vi "gmmregDefaultParameters.vi"(0 "D (3)":i32=3, 1 "nctrlPts":i32=3) -> (2 "param0":dbl[](array[numeric]), 3 "nscales":i32, 4 "default scales":dbl[](array[numeric]), 5 "deault lambdas":dbl[](array[numeric]))   [LabVIEW 2017]
panel:
  in  "lambda":dbl[](array[numeric])
  in  "scales":dbl[](array[numeric])=[1.0, 0.5, 0.1]
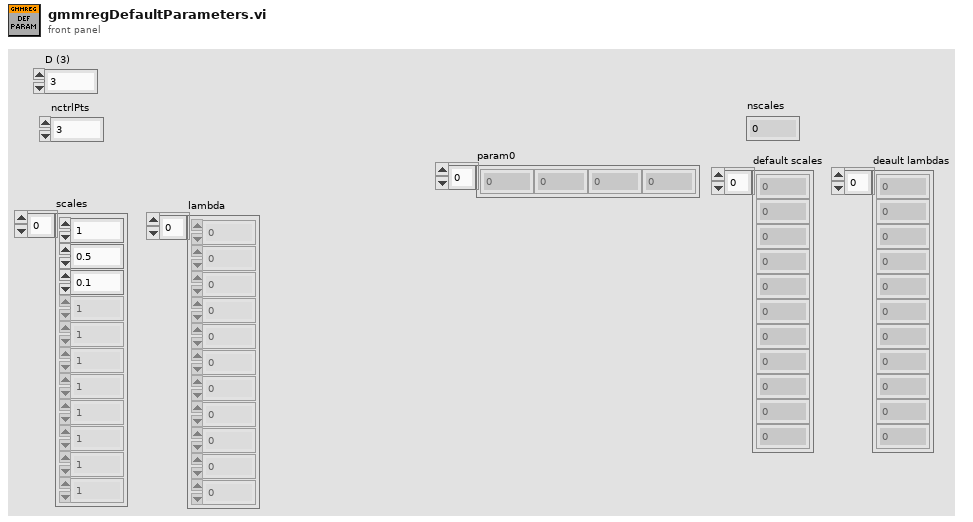
[diagram p1: front panel]
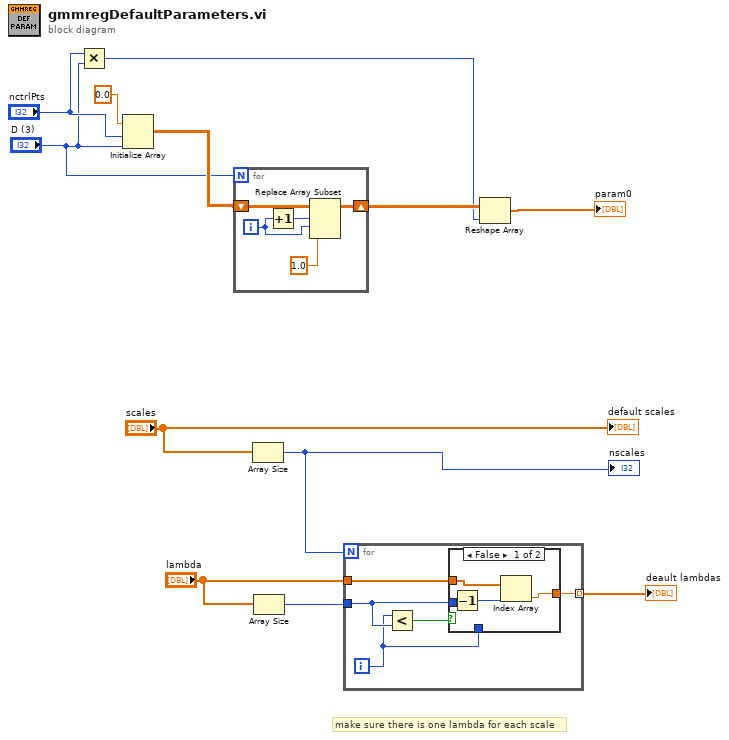
[diagram p0: block diagram]
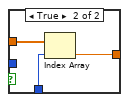
[diagram p2: hidden frame]
diagram:
  # "make sure there is one lambda for each scale"
  n1 = Multiply(x="nctrlPts", y="D (3)") -> (x*y=w2:i32)
  n2 = Initialize Array(0.0 ("element"), "nctrlPts", "D (3)") -> (w11:dbl[][])
  n3 = for {
    N: "D (3)" -> [_]
    shift-right: [w14] -> w5
    shift-left: w11 -> [w13]
    i -> [w16]
    n4 = Increment(x=w16) -> (x+1=w17:i32)
    n5 = Replace Array Subset(array=w13, new element=1.0 ("new element/subarray"), index (row)=w17, index (col)=w16) -> (w14:dbl[][])
  }
  n6 = Array Size(array="scales") -> (size(s)=w9:i32)
  "nscales" <- w9
  n7 = Array Size(array="lambda") -> (size(s)=w6:i32)
  n8 = for {
    N: w9 -> [_]
    tunnel: "lambda" -> [w22]
    tunnel: [w21] -> w8 mode=indexing
    tunnel: w6 -> [w19]
    i -> [w18]
    n9 = Less?(x=w18, y=w19) -> (x < y?=w20:bool)
    n10 = case shown="False" w20 {
      tunnel: w22 -> [w26 w29]
      tunnel: [w25 w28] -> w21
      tunnel: w19 -> [w23 _]
      tunnel: w18 -> [_ w27]
      frame False {
        n11 = Decrement(x=w23) -> (x-1=w24:i32)
        n12 = Index Array(array=w26, index=w24) -> (element=w25:dbl)
      }
      frame True {
        n13 = Index Array(array=w29, index=w27) -> (element=w28:dbl)
      }
    }
  }
  "deault lambdas" <- w8
  n14 = Reshape Array(w5, w2) -> (→"param0":dbl[])
  "default scales" <- "scales"
